vi "Read LQR Tuning.vi"(8 "error in (no error)":errorcluster, 11 "Supervisor in":refnum<class "Supervisor.lvclass">) -> (0 "error out":errorcluster, 2 "LQR Tuning":T2, 3 "Supervisor out":refnum<class "Supervisor.lvclass">)   [LabVIEW 2014, in "Supervisor.lvclass"]
uses:
  Supervisor.lvclass
  <vilib>/Analysis/Matrix/Datatypes/RealMatrix.ctl
  Supervisor.lvclass/Supervisor.ctl
  <vilib>/Analysis/Matrix/NI_Matrix.lvlib
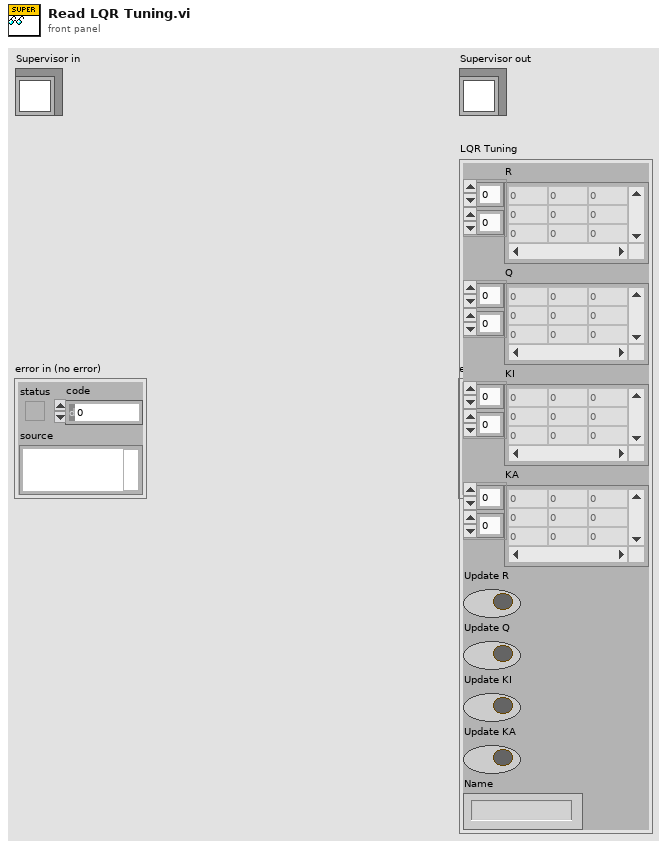
[diagram p1: front panel]
types:
  T1 = typedef "NI_Matrix.lvlib/RealMatrix.ctl" = dbl[][]
  T2 = cluster{"R":T1, "Q":T1, "KI":T1, "KA":T1, "Update R":bool, "Update Q":bool, "Update KI":bool, "Update KA":bool, "Name":string}
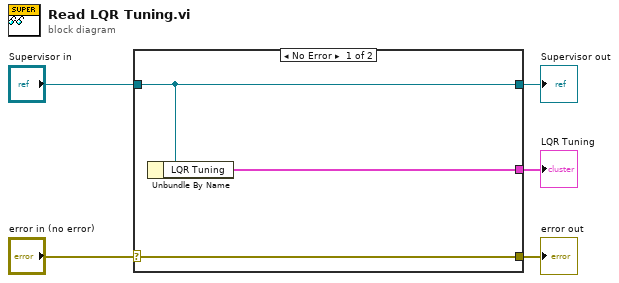
[diagram p0: block diagram]
diagram:
  n1 = case shown="No Error" "error in (no error)" {
    selector: "error in (no error)" -> [w8 w9]
    tunnel: [w8 w9] -> w4
    tunnel: [w7 w10] -> w2
    tunnel: "Supervisor in" -> [w7 w10]
    tunnel: [w6 _] -> w1
    frame No Error {
      n2 = Unbundle By Name(w7) -> ("LQR Tuning"=w6:T2)
    }
    frame Error {
    }
  }
  "error out" <- w4
  "Supervisor out" <- w2
  "LQR Tuning" <- w1
